vi "SetupDAQClock.vi"(8 "error in":errorcluster, 11 "task/channels in":refnum<k21>="Frequency1") -> (0 "error out":errorcluster, 3 "task out":refnum<k21>)   [LabVIEW 2017, in "AODControl.lvlib"]
uses:
  AODControl.lvlib
  <vilib>/DAQmx/write.llb/DAQmx Write (Digital 2D U32 NChan NSamp).vi
  <vilib>/DAQmx/configure/timing.llb/DAQmx Timing (Sample Clock).vi
  CodifyFrequency(Array).vi
  <vilib>/DAQmx/miscellaneous.llb/DAQmx Fill In Error Info.vi
  <resource>/objmgr/daqmx.rc
panel:
  out "number of samples written per channel":u32
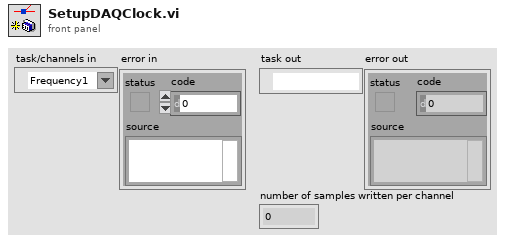
[diagram p1: front panel]
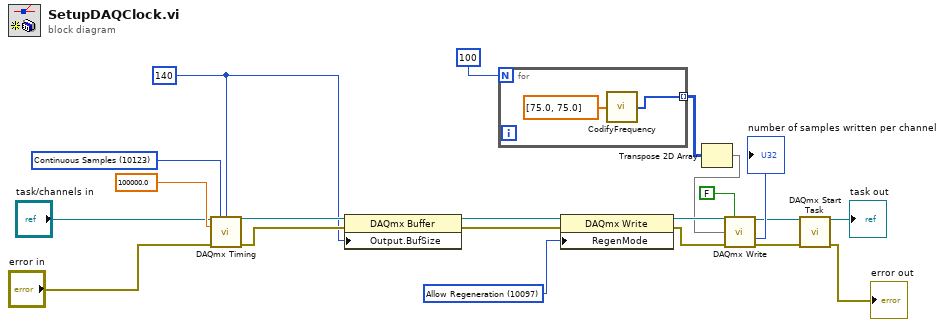
[diagram p0: block diagram]
diagram:
  w16 = 10097 items=["Allow Regeneration"=10097, "Do Not Allow Regeneration"=10158] ("RegenMode")
  w2 = 140 ("samples per channel")
  w20 = 10123 items=["Finite Samples"=10178, "Continuous Samples"=10123, "Hardware Timed Single Point"=12522] ("sample mode")
  n1 = call-poly <vilib>:"DAQmx Timing.vi"("task/channels in"="task/channels in", "sample mode"=w20, "samples per channel"=w2, "rate"=100000.0, "error in"="error in") -> ("task out"=w6:refnum<k21>, "error out"=w5:errorcluster)  [unwired: 9 in]
  n2 = property class="DAQmx Buffer"(reference=w6, error in=w5, "Output.BufSize"=w2) -> (reference out=w3:refnum<k21>, error out=w4:errorcluster)
  n3 = for {
    N: 100 -> [_]
    tunnel: [w22] -> w8 mode=indexing
    n4 = call-poly "CodifyFrequency.vi"("Array"=dbl[] [75.0, 75.0]) -> ("Array 2"=w22:u32[])
  }
  n5 = property class="DAQmx Write"(reference=w3, error in=w4, "RegenMode"=w16) -> (reference out=w17:refnum<k21>, error out=w11:errorcluster)
  n6 = Transpose 2D Array(2D array=w8) -> (transposed array=w7:u32[][])
  n7 = call-poly <vilib>:"DAQmx Write.vi"("task/channels in"=w17, "auto start"=FALSE, "data"=w7, "error in"=w11) -> ("task out"=w13:refnum<k21>, "number of samples written per channel"=→"number of samples written per channel":u32, "error out"=w10:errorcluster)  [unwired: 9 in]
  n8 = call <vilib>:"DAQmx Start Task.vi"("task/channels in"=w13, "error in"=w10) -> ("task out"=→"task out":refnum<k21>, "error out"=→"error out":errorcluster)  [unwired: 12 in]
